vi "Evaluate Part 1.vi"() -> ()   [LabVIEW 2020]
uses:
  dd8030c9-6e63-4cc6-9acf-0d191c90beec.vi
  dd8030c9-6e63-4cc6-9acf-0d191c90beec.vi/0ef24ca0-c7f0-4e73-81b6-d4fe6aada9a9.vi
  dd8030c9-6e63-4cc6-9acf-0d191c90beec.vi/0ef24ca0-c7f0-4e73-81b6-d4fe6aada9a9.vi/19e2e4cb-e3bb-4239-bd5f-680916605f5d.vi
  dd8030c9-6e63-4cc6-9acf-0d191c90beec.vi/0ef24ca0-c7f0-4e73-81b6-d4fe6aada9a9.vi/f72612c1-738a-48a1-9fcf-3db66cb27fb3.vi
  dd8030c9-6e63-4cc6-9acf-0d191c90beec.vi/0ef24ca0-c7f0-4e73-81b6-d4fe6aada9a9.vi/45406051-8994-464b-8b47-ac12a8cbadfa.vi
  dd8030c9-6e63-4cc6-9acf-0d191c90beec.vi/0ef24ca0-c7f0-4e73-81b6-d4fe6aada9a9.vi/dd886480-778c-48b1-8e4a-d6890e1a60dd.vi
  dd8030c9-6e63-4cc6-9acf-0d191c90beec.vi/0ef24ca0-c7f0-4e73-81b6-d4fe6aada9a9.vi/2e6e140f-e361-4312-a09e-e37273ac7fd1.vi
  dd8030c9-6e63-4cc6-9acf-0d191c90beec.vi/0ef24ca0-c7f0-4e73-81b6-d4fe6aada9a9.vi/3589548e-4c68-4568-af05-72ab28470577.vi
  dd8030c9-6e63-4cc6-9acf-0d191c90beec.vi/0ef24ca0-c7f0-4e73-81b6-d4fe6aada9a9.vi/cf64d4f5-91bd-4749-9577-68c6ded0155b.vi
  dd8030c9-6e63-4cc6-9acf-0d191c90beec.vi/0ef24ca0-c7f0-4e73-81b6-d4fe6aada9a9.vi/6f6fefe9-f25b-4595-b26f-75715299a794.vi
  dd8030c9-6e63-4cc6-9acf-0d191c90beec.vi/0ef24ca0-c7f0-4e73-81b6-d4fe6aada9a9.vi/c74ffb76-1048-4639-9a95-b6de96ba7014.vi
  Hand/Less Than.vi
  <vilib>/Comparison/Less/Less Functor/Less Functor.lvclass
  Hand/Hand.lvclass
panel:
  out "sum":u64
  in  "Input":string="32T3K 765\nT55J5 684\nKK677 28\nKTJJT 220\nQQQJA 483"
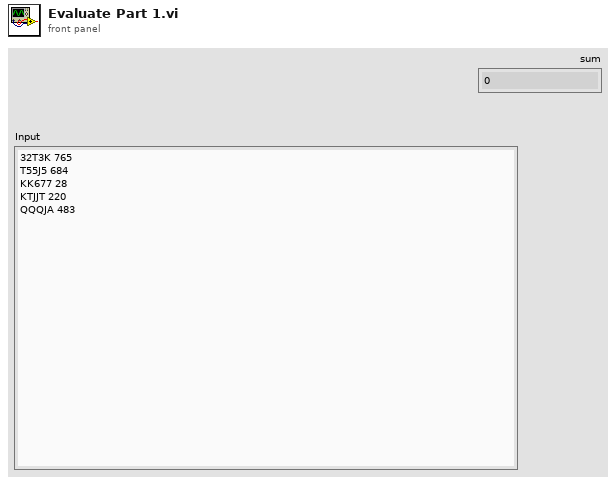
[diagram p1: front panel]
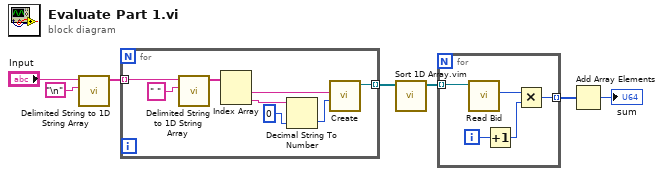
[diagram p0: block diagram]
diagram:
  n1 = call <vilib>:"Delimited String to 1D String Array.vi"("delimiter"="\n", "delimited string"="Input") -> ("string array"=w5:string[])  [unwired: 9 in]
  n2 = for {
    tunnel: w5 -> [w15] mode=indexing
    tunnel: [w8] -> w4 mode=indexing
    n3 = call <vilib>:"Delimited String to 1D String Array.vi"("delimiter"=" ", "delimited string"=w15) -> ("string array"=w13:string[])  [unwired: 9 in]
    n4 = Index Array(array=w13) -> (element #1=w10:string, element #2=w12:string)  [unwired: 2 in]
    n5 = Decimal String To Number(string=w12, default (0L)=u64 0 ("default (0 I32)")) -> (number=w9:u64)  [unwired: 1 in, 1 out]
    n6 = call "Create.vi"("Bid"=w9, "Input"=w10) -> ("Hand"=w8:refnum<class "Hand.lvclass">)  [unwired: 8 in, 1 out]
  }
  n7 = call "Sort 1D Array.vim"("unsorted array"=w4) -> ("sorted array"=w3:refnum<class "Hand.lvclass">[])  [unwired: 10 in]
  n8 = for {
    tunnel: w3 -> [w20] mode=indexing
    tunnel: [w16] -> w2 mode=indexing
    i -> [w19]
    n9 = call-dynamic "Read Bid.vi"("Hand in"=w20) -> ("Bid"=w18:u64)  [unwired: 8 in, 2 out]
    n10 = Increment(x=w19) -> (x+1=w17:i32)
    n11 = Multiply(x=w18, y=w17) -> (x*y=w16:u64)
  }
  n12 = Add Array Elements(numeric array=w2) -> (sum=→"sum":u64)
